vi "testing_checksum_error_32-bit.vi"() -> ()   [LabVIEW 2015, in "Tausand AB1000.lvlib"]
uses:
  <instrlib>/Tausand AB1000/Tausand AB1000.lvlib
  <instrlib>/Tausand AB1000/Public/Controls/serialCommand.ctl
panel:
  in  "numtests":i32=10000 caption="Number of tests"
  out "checksum error percentage":dbl(slide) scale=0.0..100.0
  out "error out":errorcluster
  out "bytes read":u32
  out "data32 out":u32[](array[numeric])
  out "number of errors":i16
  out "i":i32 caption="test number"
  in  "VISA resource name":refnum<visa-resource-name>
  out "hist chks":bool[](array[boolean]) caption="Historic of checksum"
  in  "stop":bool
  # "CheckSumError rate test\nFor 32-bit devices\nDavid Guzman, June 2021"
  # "Current read"
  # "Checksum error report"
  # "of"
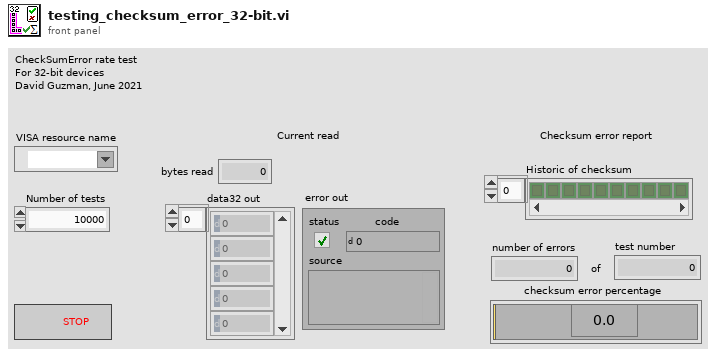
[diagram p1: front panel]
types:
  T1 = typedef "Tausand AB1000.lvlib/serialCommand.ctl" = u8
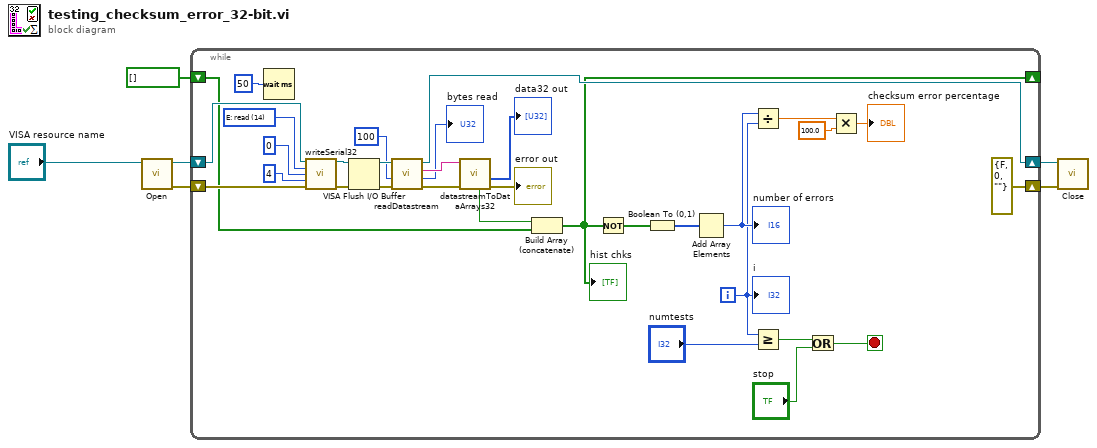
[diagram p0: block diagram]
diagram:
  n1 = call <instrlib>:"Open.vi"("VISA resource name"="VISA resource name") -> ("error out"=w3:errorcluster, "VISA resource name out"=w6:refnum<visa-resource-name>)  [unwired: 9 in]
  n2 = while {
    shift-right: [w36] -> w5
    shift-left: w6 -> [w29]
    shift-right: [errorcluster {"status"=FALSE, "code"=0, "source"=""} ("error out")] -> w4
    shift-left: w3 -> [w28]
    shift-right: [w12] -> _
    shift-left: bool[] [] -> [w13]
    i -> [w11]
    stop <- w7 stop-if-true
    w32 = T1 14 items=["0", "1", "2", "3", "4", "5", "6", "7", "8", "9", "A", "B", "C", "D", "E: read", "F: write"] ("command (E: read)")
    n3 = Wait (ms)(milliseconds to wait=u32 50) -> ()  [unwired: 1 out]
    n4 = call <instrlib>:"writeSerial32.vi"("VISA Refnum in"=w29, "command (E: read)"=w32, "address"=u8 0, "data U32 (0)"=u32 4, "error in (no error)"=w28) -> ("VISA Refnum out"=w27:refnum<visa-resource-name>, "error out"=w24:errorcluster)  [unwired: 9 in]
    n5 = VISA Flush I/O Buffer(VISA resource name=w27, error in (no error)=w24) -> (VISA resource name out=w26:refnum<visa-resource-name>, error out=w25:errorcluster)  [unwired: 1 in]
    n6 = call <instrlib>:"readDatastream.vi"("error in (no error)"=w25, "Timeout (10000 ms)"=u32 100, "VISA Refnum in"=w26) -> ("error out"=w38:errorcluster, "bytes read"=→"bytes read":u32, "string out"=w37:string, "VISA Refnum out"=w36:refnum<visa-resource-name>)  [unwired: 4 in, 1 out]
    n7 = call <instrlib>:"datastreamToDataArrays32.vi"("error in (no error)"=w38, "input string"=w37) -> ("error out"=→"error out":errorcluster, "data32 out"=→"data32 out":u32[], "checksum ok"=w14:bool)  [unwired: 5 in, 2 out]
    n8 = Build Array (concatenate)(w14, w13) -> (w12:bool[])
    "hist chks" <- w12
    n9 = Not(x=w12) -> (.not. x?=w19:bool[])
    n10 = Boolean To (0,1)(Boolean=w19) -> (0, 1=w34:i16[])
    n11 = Add Array Elements(numeric array=w34) -> (sum=w18:i16)
    "number of errors" <- w18
    n12 = Divide(x=w18, y=w11) -> (x/y=w17:dbl)
    n13 = Greater Or Equal?(x=w11, y="numtests") -> (x >= y?=w8:bool)
    n14 = Or(x=w8, y="stop") -> (x .or. y?=w7:bool)
    n15 = Multiply(x=w17, y=100.0) -> (x*y=→"checksum error percentage":dbl)
    "i" <- w11
  }
  n16 = call <instrlib>:"Close.vi"("error in (no error)"=w4, "VISA resource name"=w5) -> ()  [unwired: 9 in, 1 out]
